vi "ev3-gamepad.vi"() -> ()   [LabVIEW 2013]
uses:
  <vilib>/Utility/inputDevices.llb/closeJoystick.vi
  <vilib>/Utility/inputDevices.llb/joystickAcquire.vi
panel:
  out "mouse info":T1(array[cluster])
  out "key info":T2(array[cluster])
  out "joystick info":T3(array[cluster])
  in  "device index":i32
  in  "stop":bool
  out "button info":T4
  out "axis info":T5
  out "direction info":T6
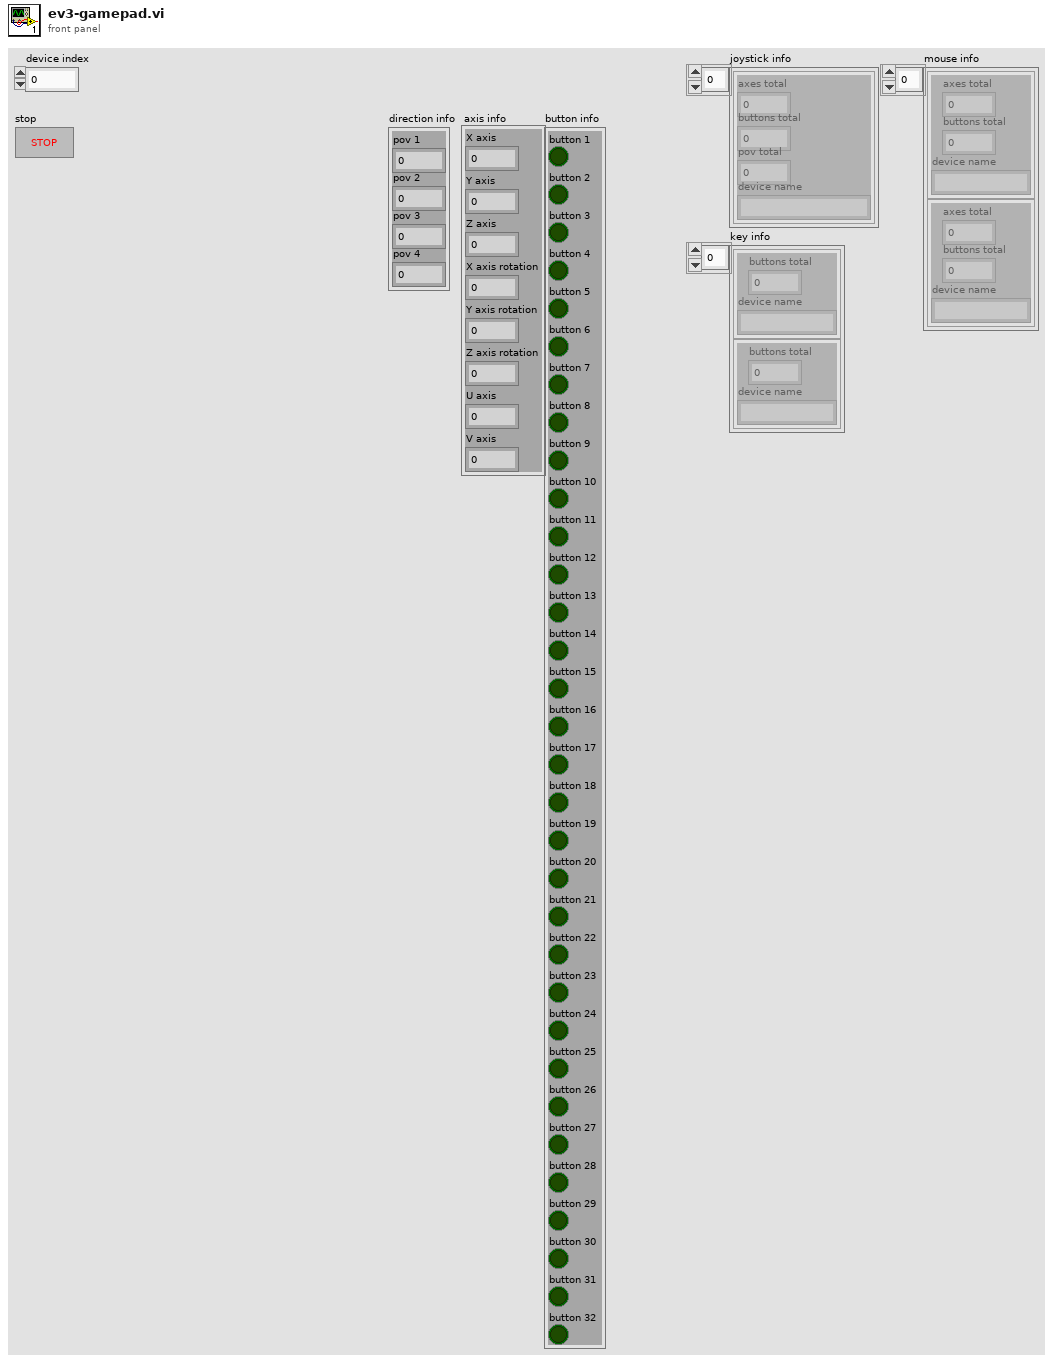
[diagram p1: front panel]
types:
  T1 = cluster{"axes total":u32, "buttons total":u32, "device name":string}[]
  T2 = cluster{"buttons total":u32, "device name":string}[]
  T3 = cluster{"axes total":u32, "buttons total":u32, "pov total":u32, "device name":string}[]
  T4 = cluster{"button 1":bool, "button 2":bool, "button 3":bool, "button 4":bool, "button 5":bool, "button 6":bool, "button 7":bool, "button 8":bool, "button 9":bool, "button 10":bool, "button 11":bool, "button 12":bool, "button 13":bool, "button 14":bool, "button 15":bool, "button 16":bool, "button 17":bool, "button 18":bool, "button 19":bool, "button 20":bool, "button 21":bool, "button 22":bool, "button 23":bool, "button 24":bool, "button 25":bool, "button 26":bool, "button 27":bool, "button 28":bool, "button 29":bool, "button 30":bool, "button 31":bool, "button 32":bool}
  T5 = cluster{"X axis":i32, "Y axis":i32, "Z axis":i32, "X axis rotation":i32, "Y axis rotation":i32, "Z axis rotation":i32, "U axis":i32, "V axis":i32}
  T6 = cluster{"pov 1":i32, "pov 2":i32, "pov 3":i32, "pov 4":i32}
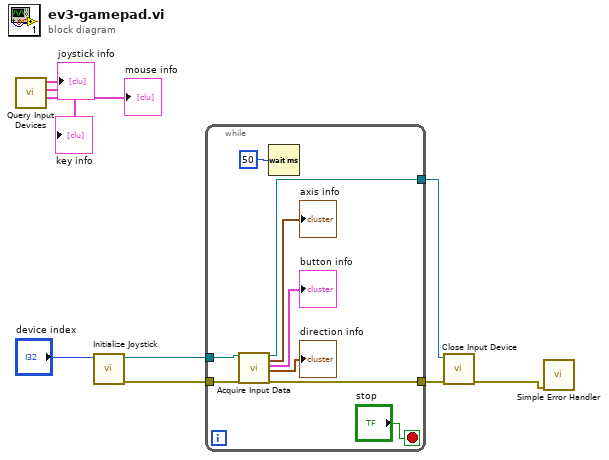
[diagram p0: block diagram]
diagram:
  n1 = call <vilib>:"Query Input Devices.vi"() -> ("mouse info"=→"mouse info":T1, "key info"=→"key info":T2, "joystick info"=→"joystick info":T3)  [unwired: 8 in, 1 out]
  n2 = call <vilib>:"Initialize Joystick.vi"("device index"="device index") -> ("error out"=w7:errorcluster, "device ID"=w9:refnum<k1>)  [unwired: 9 in]
  n3 = while {
    tunnel: w9 -> [w18]
    tunnel: [w17] -> w8
    tunnel: w7 -> [w16]
    tunnel: [w15] -> w6
    stop <- "stop" stop-if-true
    n4 = call-poly <vilib>:"Acquire Input Data.vi"("device ID"=w18, "error in (no error)"=w16) -> ("device ID"=w17:refnum<k1>, "axis info"=→"axis info":T5, "button info"=→"button info":T4, "direction info"=→"direction info":T6, "error out"=w15:errorcluster)  [unwired: 13 in]
    n5 = Wait (ms)(milliseconds to wait=u32 50) -> ()  [unwired: 1 out]
  }
  n6 = call-poly <vilib>:"Close Input Device.vi"("error in (no error)"=w6, "device ID"=w8) -> ("error out"=w3:errorcluster)  [unwired: 8 in]
  n7 = call <vilib>:"Simple Error Handler.vi"("error in (no error)"=w3) -> ()  [unwired: 4 in, 5 out]
